vi "Actor Core.vi"(8 "error in (no error)":errorcluster, 11 "Common Measurements Interface in":refnum<class "Common Measurements Interface.lvclass">) -> (0 "error out":errorcluster, 3 "Actor Framework.lvlib:Actor":refnum<class "Actor.lvclass">)   [LabVIEW 2015, in "Common Measurements Interface.lvclass"]
uses:
  Common Measurements Interface.lvclass
  <vilib>/ActorFramework/Actor/Actor.lvclass
  Queued Listbox/Queued Listbox.xctl
  Common Measurements Interface.lvclass/Common Measurements Interface.ctl
  Mag Lab Measure Interface/Mag Lab Measure UI.lvclass/Mag Lab Measure UI.ctl
  <vilib>/ActorFramework/Actor/Actor.lvclass/Actor.ctl
  <vilib>/ActorFramework/Message Enqueuer/Message Enqueuer.lvclass/Message Enqueuer.ctl
  Mag Lab Graph/MagLabGraph.lvclass
  Mag Lab Measure Base Messages/Launch graph Msg/Launch graph Msg.lvclass/Launch graph Msg.ctl
  Mag Lab Root Messages/Write CFG File Msg/Write CFG File Msg.lvclass/Write CFG File Msg.ctl
  Mag Lab Root Messages/Read CFG File Msg/Read CFG File Msg.lvclass/Read CFG File Msg.ctl
  Mag Lab Measure Controller Messages/Start measurements Msg/Start measurements Msg.lvclass/Start measurements Msg.ctl
  Mag Lab Measure Controller Messages/Pause measurements Msg/Pause measurements Msg.lvclass/Pause measurements Msg.ctl
  <vilib>/ActorFramework/Message Enqueuer/Init from Existing Queue.vi
  <vilib>/ActorFramework/Message Enqueuer/Enqueue.vi
  <vilib>/ActorFramework/Message Priority Queue/Priority Enqueue.vi
  <vilib>/ActorFramework/Message Enqueuer/Message Enqueuer.lvclass
  <vilib>/ActorFramework/Stop Msg/Stop Msg.lvclass
  Mag Lab Measure Base Messages/Launch graph Msg/Launch graph Msg.lvclass
  Mag Lab Root Messages/Write CFG File Msg/Write CFG File Msg.lvclass
  Mag Lab Root Messages/Read CFG File Msg/Read CFG File Msg.lvclass
  Mag Lab Measure Controller Messages/Start measurements Msg/Start measurements Msg.lvclass
  Mag Lab Measure Controller Messages/Pause measurements Msg/Pause measurements Msg.lvclass
  Mag Lab Measure Controller Messages/Stop all measurements Msg/Stop all measurements Msg.lvclass
  Mag Lab Measure Interface/Interface with menu/Interface with menu.lvclass
  Mag Lab Measure Interface/Mag Lab Measure UI.lvclass
  Mag Lab Error Handler/Mag Lab Error Handler.lvclass
panel:
  out "Running":bool
  in  "Parameters":T1={"Syncronize measurements "=FALSE, "Repeat times"=-1}
  in  "Write cfg":bool
  in  "Read cfg":bool
  in  "Pause":bool
  in  "Time Stamp":timestamp
  in  "Stop":bool
  out "File Path":path
  in  "Graph":bool
  in  "Run":bool
  in  "Measure":string[](xcontrol)
  out "Name":string
  in  "Parameters":cluster{"Text":string}
  out "Log":string
  in  "Exit":bool
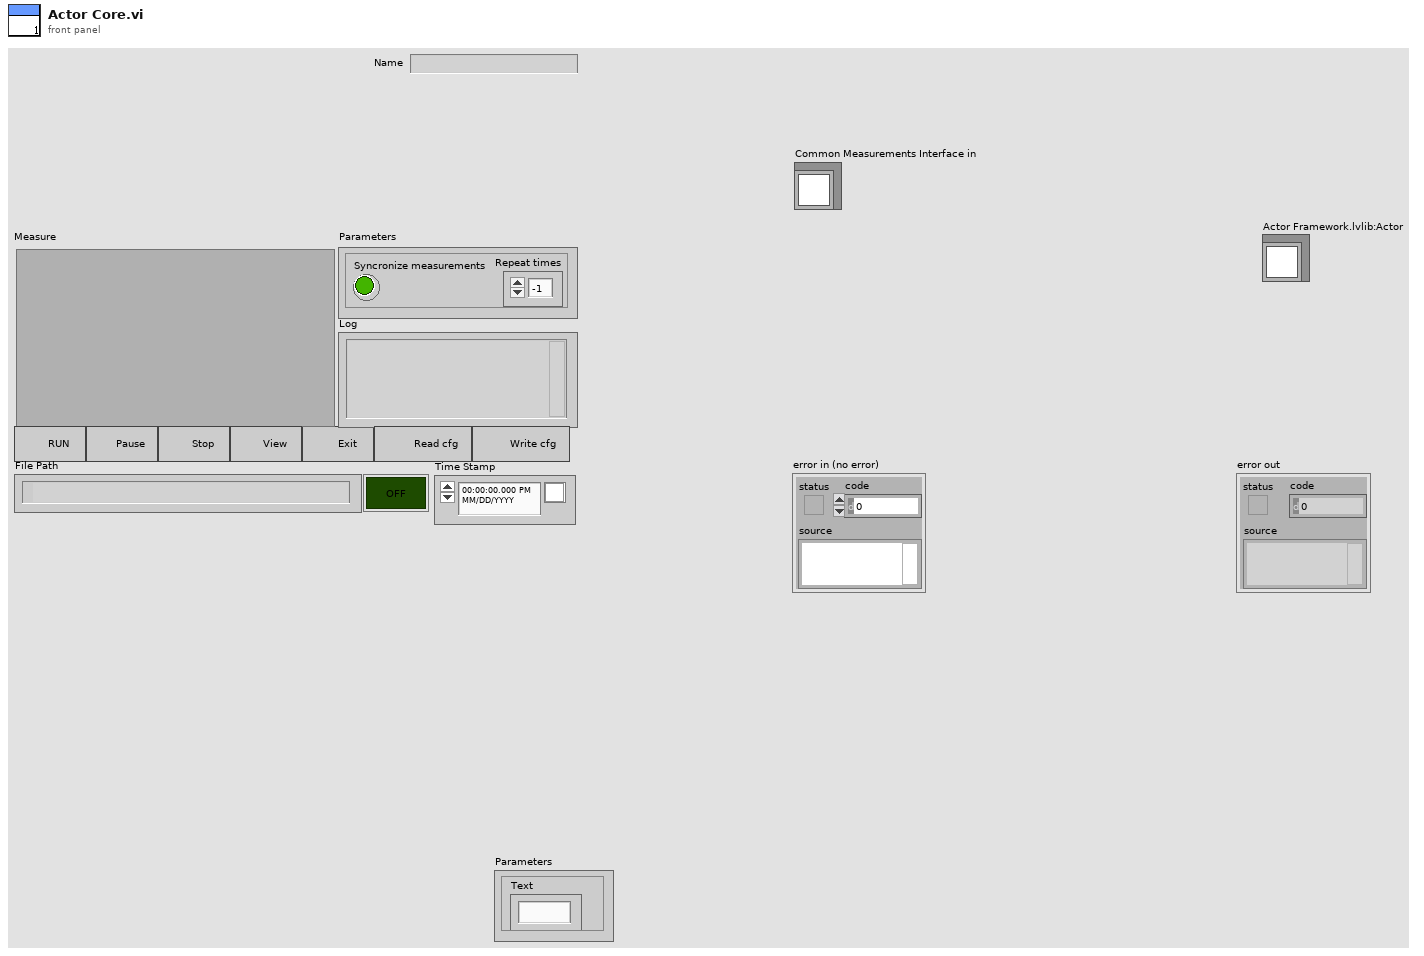
[diagram p1: front panel]
types:
  T1 = cluster{"Syncronize measurements ":bool, "Repeat times":i32}
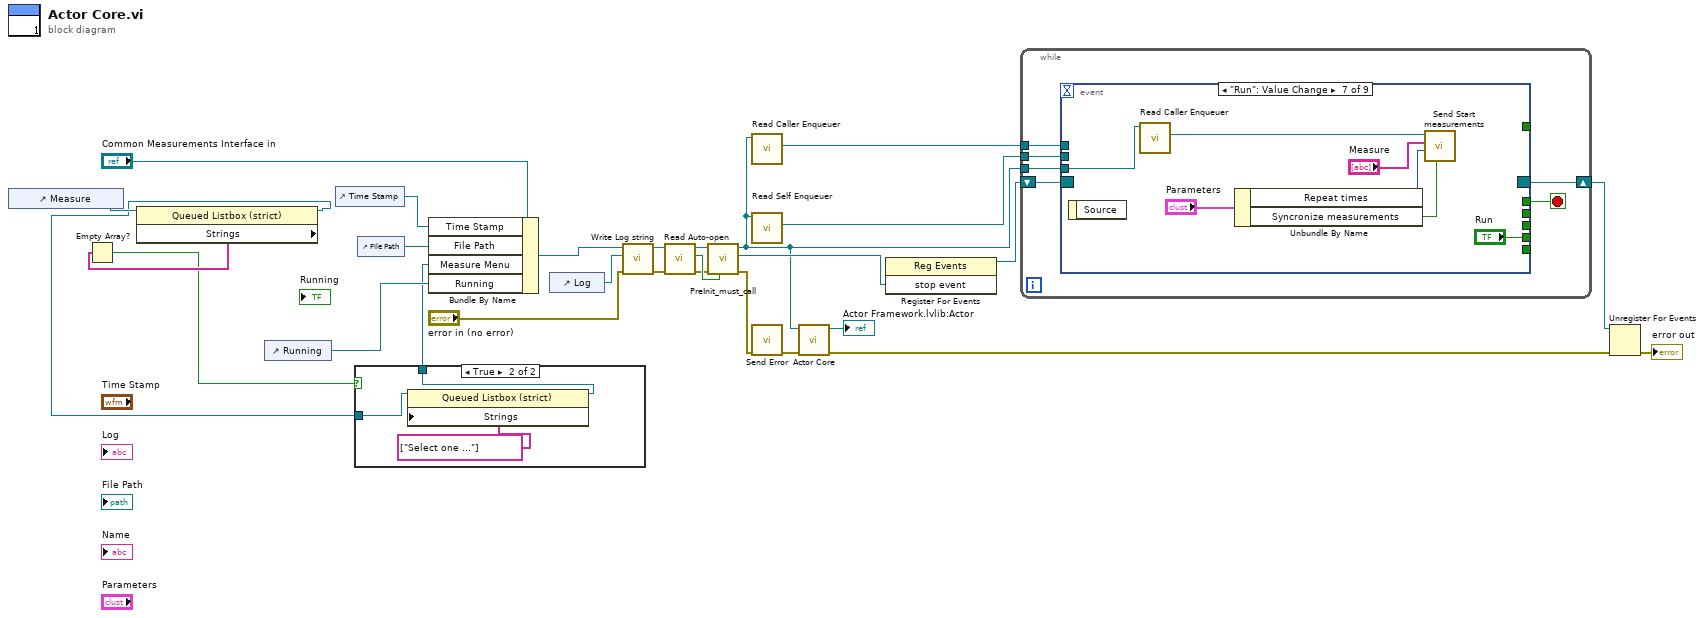
[diagram p0: block diagram]
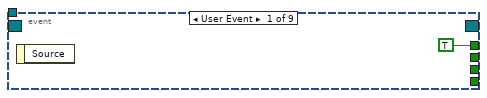
[diagram p3: hidden frame]
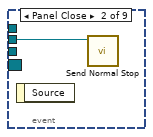
[diagram p4: hidden frame]
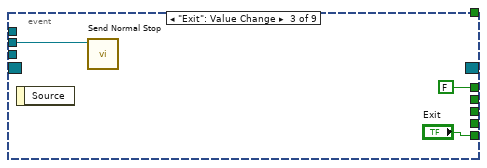
[diagram p5: hidden frame]
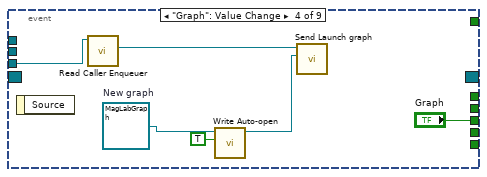
[diagram p6: hidden frame]
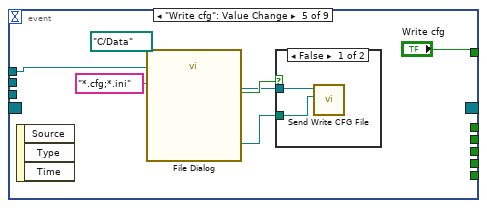
[diagram p7: hidden frame]
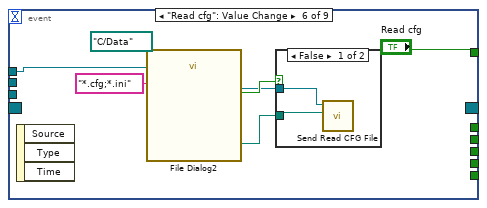
[diagram p9: hidden frame]
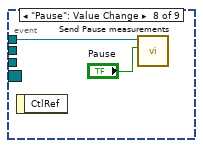
[diagram p11: hidden frame]
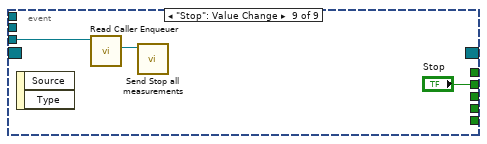
[diagram p12: hidden frame]
diagram:
  n1 = control-ref of="Measure"() -> (w19:refnum<vi>)
  n2 = property class="Queued Listbox (strict)"(reference=w19) -> (reference out=w2:refnum<vi>, "Strings"=w4:string[])  [unwired: 1 in, 1 out]
  n3 = Empty Array?(array=w4) -> (empty?=w3:bool)
  n4 = control-ref of="Running"() -> (w5:refnum<vi>)
  n5 = control-ref of="Time Stamp"() -> (w13:refnum<vi>)
  n6 = case shown="True" w3 {
    tunnel: w2 -> [w29 w32]
    tunnel: [w29 w31] -> w1
    frame False {
    }
    frame True {
      n7 = property class="Queued Listbox (strict)"(reference=w32, "Strings"=string[] ["Select one ..."]) -> (reference out=w31:refnum<vi>)  [unwired: 1 in, 1 out]
    }
  }
  n8 = control-ref of="File Path"() -> (w14:refnum<vi>)
  n9 = Bundle By Name(cluster="Common Measurements Interface in", "Time Stamp"=w13, "File Path"=w14, "Measure Menu"=w1, "Running"=w5) -> (w20:refnum<class "Common Measurements Interface.lvclass">)
  n10 = control-ref of="Log"() -> (w25:refnum<vi>)
  n11 = call "Write Log string.vi"("error in (no error)"="error in (no error)", "Log string"=w25, "Mag Lab Measure Interface in"=w20) -> ("error out"=w9:errorcluster, "Mag Lab Measure Interface out"=w12:refnum<class "Common Measurements Interface.lvclass">)  [unwired: 7 in]
  n12 = call "Read Auto-open.vi"("error in (no error)"=w9, "Mag Lab Measure UI in"=w12) -> ("error out"=w8:errorcluster, "Auto-open"=w10:bool, "Mag Lab Measure UI out"=w11:refnum<class "Common Measurements Interface.lvclass">)  [unwired: 7 in]
  n13 = call-dynamic "PreInit_must_call.vi"("Open Actor Core front panel? (T)"=w10, "error in (no error)"=w8, "Mag Lab Measure Interface in"=w11) -> ("error out"=w18:errorcluster, "stop event"=w26:refnum<user-event>, "Mag Lab Measure Interface out"=w7:refnum<class "Common Measurements Interface.lvclass">)  [unwired: 6 in]
  n14 = call <vilib>:"Read Caller Enqueuer.vi"("Actor"=w7) -> ("Caller Enqueuer"=w6:refnum<class "Message Enqueuer.lvclass">)  [unwired: 10 in]
  n15 = call <vilib>:"Read Self Enqueuer.vi"("Actor"=w7) -> ("Self Enqueuer"=w24:refnum<class "Message Enqueuer.lvclass">)  [unwired: 10 in]
  n16 = call "Send Error.vi"("error in (no error)"=w18) -> ("error out"=w23:errorcluster)  [unwired: 9 in, 1 out]
  n17 = call-parent "Actor Core.vi"("error in (no error)"=w23, "Mag Lab Measure Interface in"=w7) -> ("error out"=w15:errorcluster, "Actor Framework.lvlib:Actor"=→"Actor Framework.lvlib:Actor":refnum<class "Actor.lvclass">)  [unwired: 8 in]
  n18 = register-events(w26) -> (reference out=w27:refnum<event-registration>)  [unwired: 2 in, 1 out]
  n19 = while {
    tunnel: w24 -> [w36]
    shift-right: [w35] -> w16
    shift-left: w27 -> [w37]
    tunnel: w7 -> [w34]
    tunnel: w6 -> [w33]
    stop <- w38 stop-if-true
    n20 = event shown="[6] \"Run\": Value Change" {
      selector: w37 -> [_ _ _ _ _ _ _ _ _]
      dyn-events: [_ _ _ _ _ _ _ _ _] -> w35
      timeout: _ -> [_ _ _ _ _ _ _ _ _]
      tunnel: [TRUE _ FALSE _ _ _ _ _ _] -> w38
      tunnel: w36 -> [_ w40 w41 _ _ _ _ _ _]
      tunnel: [_ _ "Exit" _ _ _ _ _ _] -> _
      tunnel: [_ _ _ _ _ _ "Run" _ _] -> _
      tunnel: w34 -> [_ _ _ w49 _ _ w71 _ w76]
      tunnel: [_ _ _ "Graph" _ _ _ _ _] -> _
      tunnel: [_ _ _ _ _ _ _ _ "Stop"] -> _
      tunnel: w33 -> [_ _ _ _ w50 w59 _ w73 _]
      tunnel: [_ _ _ _ "Write cfg" "Read cfg" _ _ _] -> _
      event User Event {
        n21 = event-data() -> ()  [unwired: 1 in, 1 out]
      }
      event Panel Close {
        n22 = event-data() -> ()  [unwired: 1 in, 1 out]
        n23 = call <vilib>:"Send Normal Stop.vi"("Message Enqueuer"=w40) -> ()  [unwired: 10 in, 1 out]
      }
      event "Exit": Value Change {
        n24 = event-data() -> ()  [unwired: 1 in, 1 out]
        n25 = call <vilib>:"Send Normal Stop.vi"("Message Enqueuer"=w41) -> ()  [unwired: 10 in, 1 out]
      }
      event "Graph": Value Change {
        w46 = refnum<class "MagLabGraph.lvclass"> refnum  # New graph
        n26 = event-data() -> ()  [unwired: 1 in, 1 out]
        n27 = call <vilib>:"Read Caller Enqueuer.vi"("Actor"=w49) -> ("Caller Enqueuer"=w48:refnum<class "Message Enqueuer.lvclass">)  [unwired: 10 in]
        n28 = call "Write Auto-open.vi"("Auto-open"=TRUE, "Mag Lab Measure UI in"=w46) -> ("Mag Lab Measure UI out"=w45:refnum<class "MagLabGraph.lvclass">)  [unwired: 8 in, 1 out]
        n29 = call "Send Launch graph.vi"("MagLabGraph.lvclass"=w45, "Message Enqueuer"=w48) -> ()  [unwired: 8 in, 2 out]
      }
      event "Write cfg": Value Change {
        n30 = event-data() -> ()  [unwired: 1 in, 3 out]
        n31 = call "File Dialog"("start path"=path "C:/Data", "pattern (all files)"="*.cfg;*.ini") -> ("selected path"=w51:path, "cancelled"=w52:bool)  [unwired: 10 in, 2 out]
        n32 = case shown="False" w52 {
          tunnel: w50 -> [w57 _]
          tunnel: w51 -> [w56 _]
          frame False {
            n33 = call "Send Write CFG File.vi"("File path"=w56, "Message Enqueuer"=w57) -> ()  [unwired: 8 in, 2 out]
          }
          frame True {
          }
        }
      }
      event "Read cfg": Value Change {
        n34 = event-data() -> ()  [unwired: 1 in, 3 out]
        n35 = call "File Dialog2"("start path"=path "C:/Data", "pattern (all files)"="*.cfg;*.ini") -> ("selected path"=w60:path, "cancelled"=w61:bool)  [unwired: 10 in, 2 out]
        n36 = case shown="False" w61 {
          tunnel: w59 -> [w65 _]
          tunnel: w60 -> [w64 _]
          frame False {
            n37 = call "Send Read CFG File.vi"("File path"=w64, "Message Enqueuer"=w65) -> ()  [unwired: 8 in, 2 out]
          }
          frame True {
          }
        }
      }
      event "Run": Value Change {
        n38 = event-data() -> ()  [unwired: 1 in, 1 out]
        n39 = call <vilib>:"Read Caller Enqueuer.vi"("Actor"=w71) -> ("Caller Enqueuer"=w70:refnum<class "Message Enqueuer.lvclass">)  [unwired: 10 in]
        n40 = Unbundle By Name("Parameters") -> ("Repeat times"=w67:i32, "Syncronize measurements"=w66:bool)
        n41 = call "Send Start measurements.vi"("Syncronize measurements"=w66, "Repeat times"=w67, "Measurements"="Measure", "Message Enqueuer"=w70) -> ()  [unwired: 6 in, 2 out]
      }
      event "Pause": Value Change {
        n42 = event-data() -> ()  [unwired: 1 in, 1 out]
        n43 = call "Send Pause measurements.vi"("Pause"="Pause", "Message Enqueuer"=w73) -> ()  [unwired: 8 in, 2 out]
      }
      event "Stop": Value Change {
        n44 = event-data() -> ()  [unwired: 1 in, 2 out]
        n45 = call <vilib>:"Read Caller Enqueuer.vi"("Actor"=w76) -> ("Caller Enqueuer"=w75:refnum<class "Message Enqueuer.lvclass">)  [unwired: 10 in]
        n46 = call "Send Stop all measurements.vi"("Message Enqueuer"=w75) -> ()  [unwired: 9 in, 2 out]
      }
    }
  }
  n47 = Unregister For Events(event registration refnum=w16, error in=w15) -> (error out=→"error out":errorcluster)
